vi "Main.vi"() -> ()   [LabVIEW 2018]
doc: "Use this template to build a simple state machine design pattern. Each state executes code and determines which state to transition to."
uses:
  controls/State.ctl
  controls/Data.ctl
  <vilib>/Analysis/NI_AALPro.lvlib
panel:
  in  "mA":dbl=4.0 format="%.3f"
  out "Physical Value":dbl
  in  "Compute Physical Value":bool
  out "Slope":dbl
  out "Offset":dbl
  out "XY Graph":cluster{dbl[], dbl[]}(graph)
  in  "Max mA Output":dbl
  in  "Min mA Output":dbl
  in  "Max Physical Value":dbl
  in  "Min Physical Value":dbl
  in  "Completion Resistor(Ohms)":u16
  in  "Compute Coefficients":bool
  in  "Exit":bool
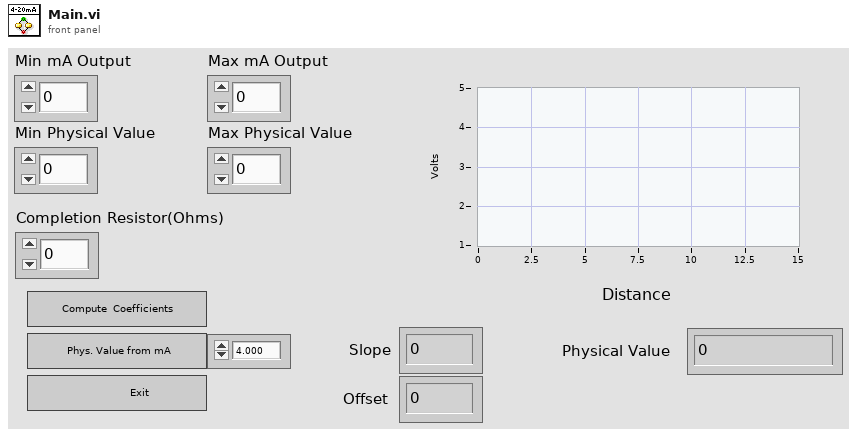
[diagram p1: front panel]
types:
  T1 = typedef "Data.ctl" = cluster{"Completion Resistor(Ohms)":dbl, "Min Physical Value":dbl, "Max Physical Value":dbl, "Min mA Output":dbl, "Max mA Output":dbl, "Measured mA Output":dbl, "Min Voltage":dbl, "Max Voltage":dbl, "m [f(x)]":dbl, "b [f(x)]":dbl, "m [f(y)]":dbl, "b [f(y)]":dbl}
  T2 = typedef "State.ctl" = enum16{"Initialize", "Wait for Event", "Compute Coefficients", "Compute MinMax Volts", "Compute f(x) Slope & Offset", "Compute f(y) Slope & Offset", "Compute Physical Value from mA", "Display Physical Value", "Exit"}
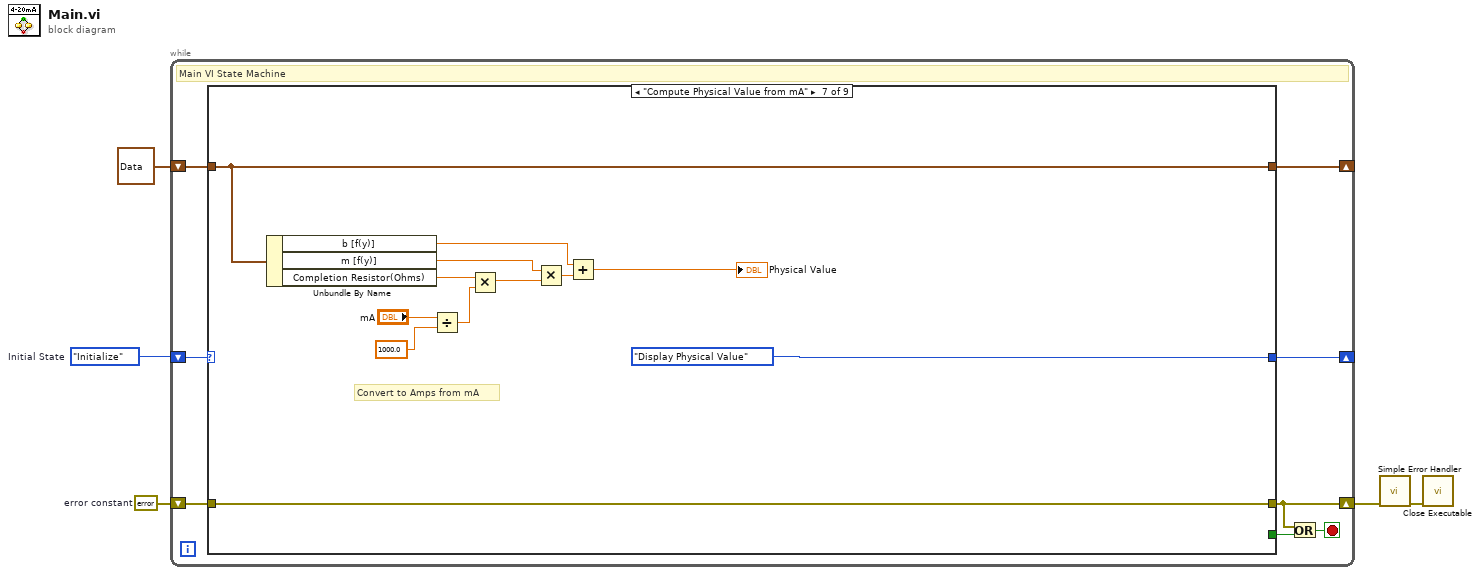
[diagram p0: block diagram]
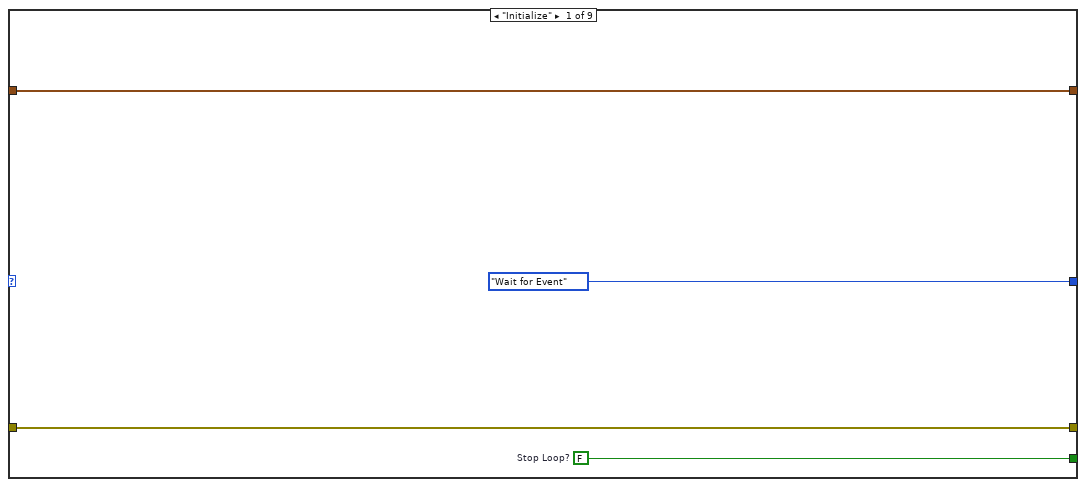
[diagram p2: hidden frame]
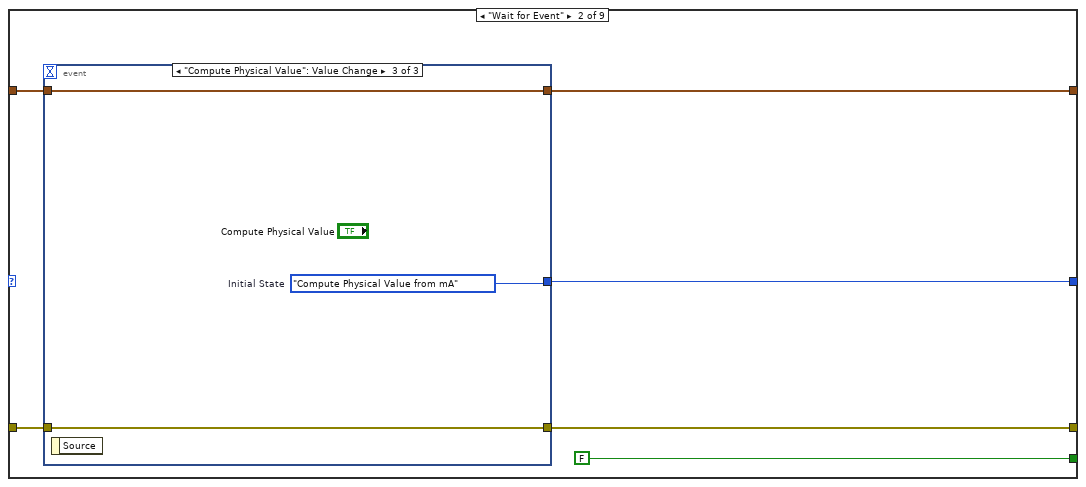
[diagram p3: hidden frame]
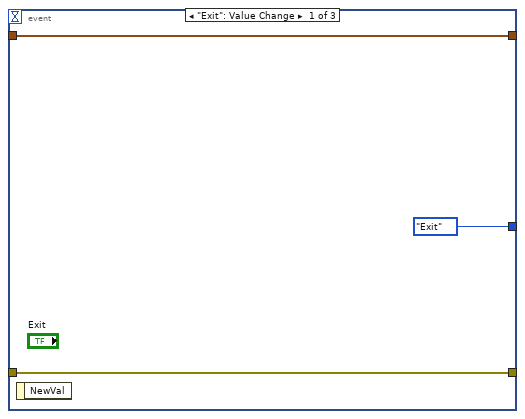
[diagram p4: hidden frame]
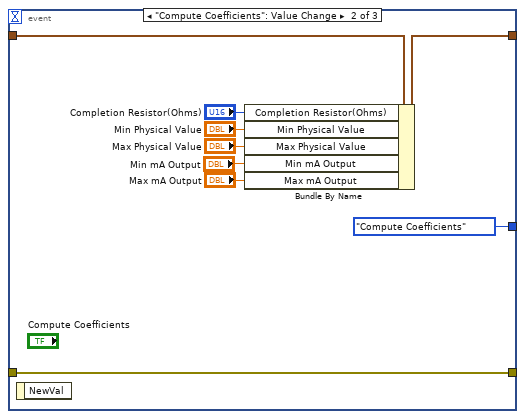
[diagram p5: hidden frame]
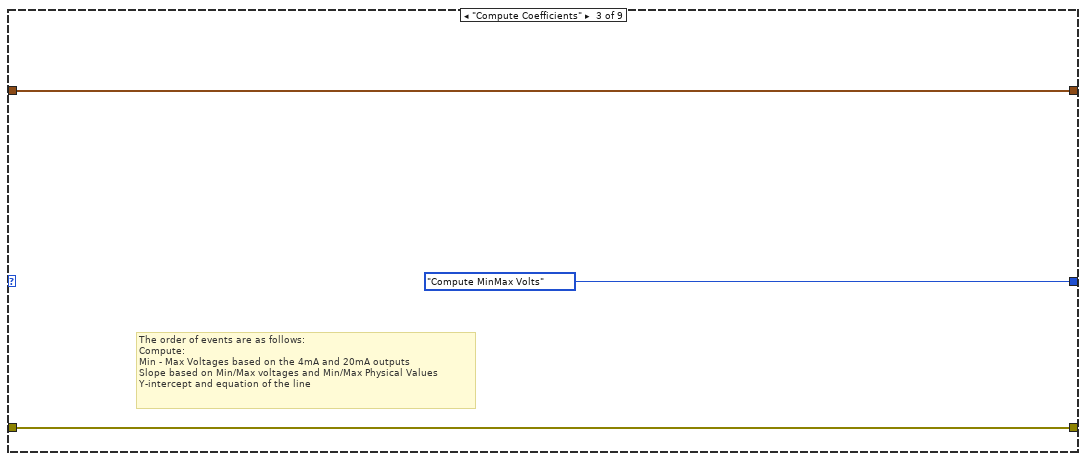
[diagram p6: hidden frame]
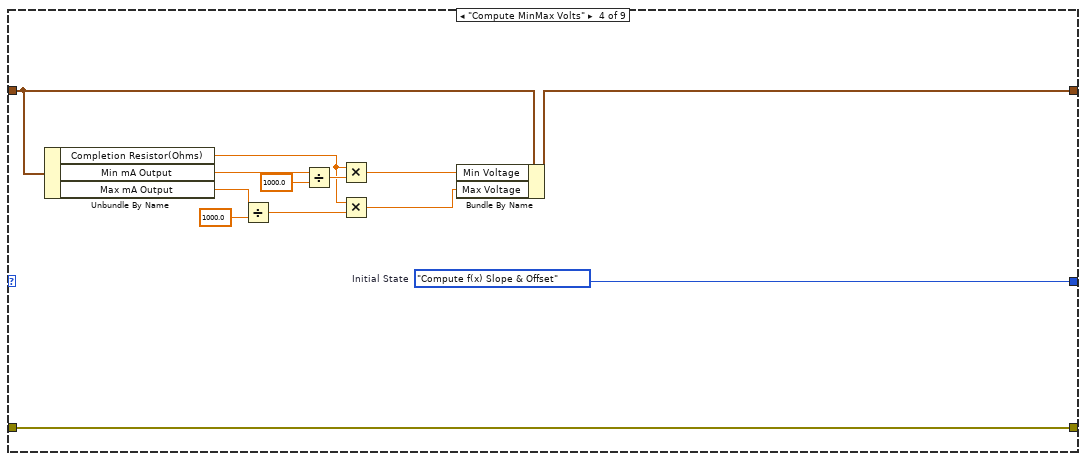
[diagram p7: hidden frame]
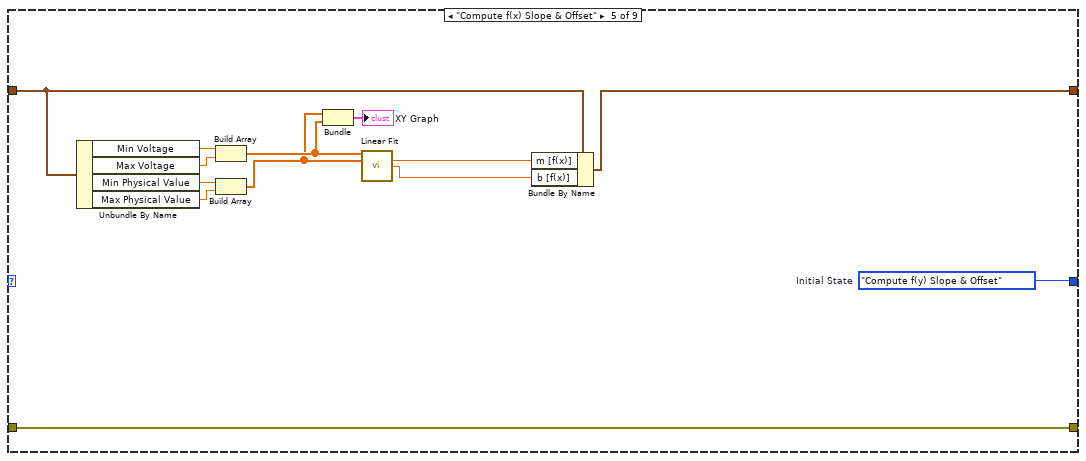
[diagram p8: hidden frame]
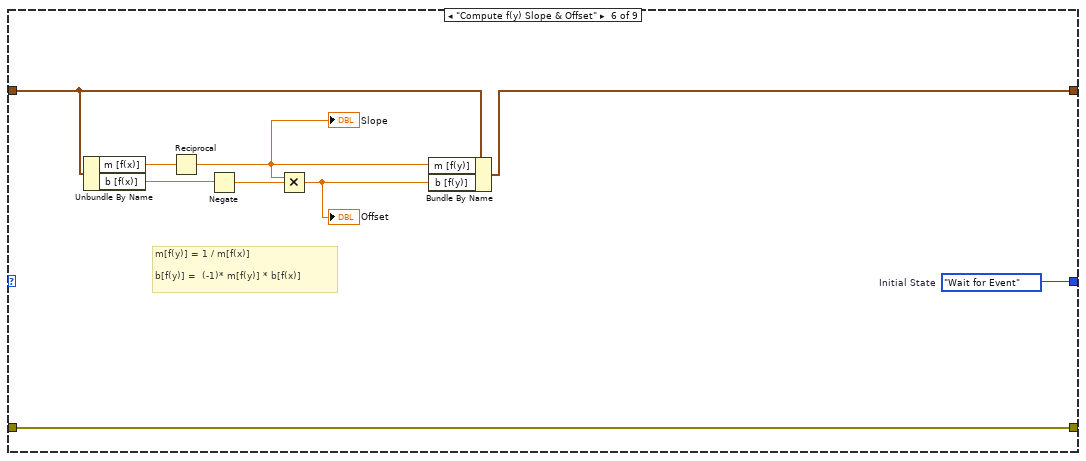
[diagram p9: hidden frame]
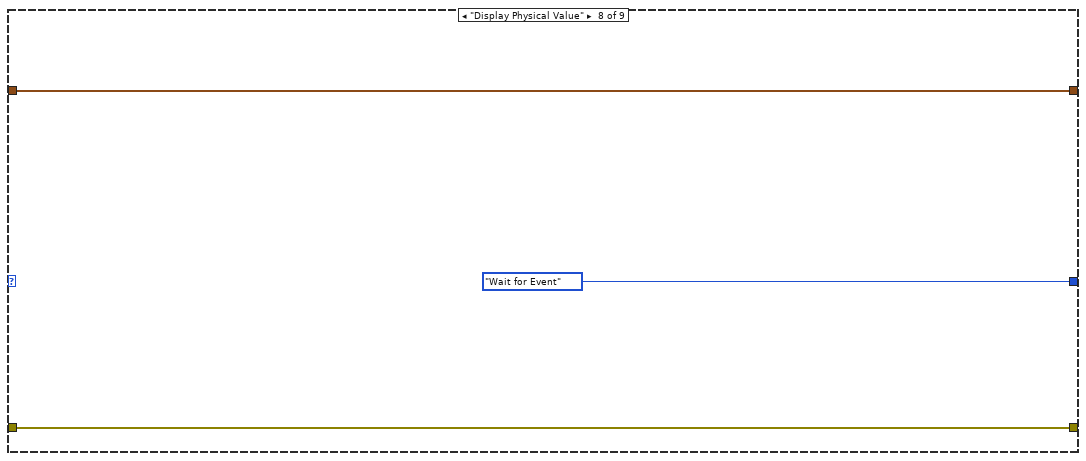
[diagram p10: hidden frame]
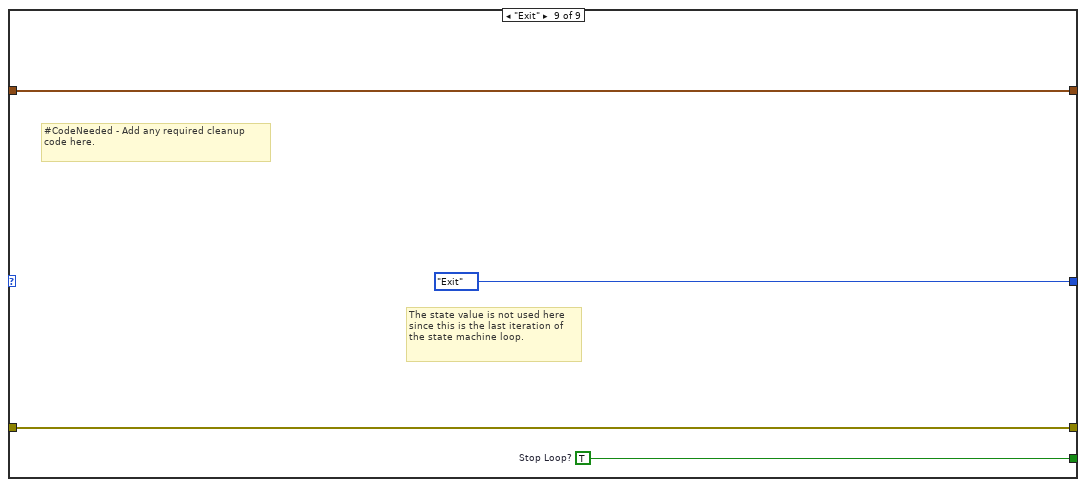
[diagram p11: hidden frame]
diagram:
  w4 = errorcluster {"status"=FALSE, "code"=0, "source"=""}  # error constant
  w1 = State."Initialize"  # Initial State
  n1 = while {
    shift-right: [w6] -> _
    shift-left: w1 -> [w7]
    shift-right: [w12] -> _
    shift-left: T1 {"Completion Resistor(Ohms)"=0.0, "Min Physical Value"=0.0, "Max Physical Value"=0.0, "Min mA Output"=0.0, "Max mA Output"=0.0, "Measured mA Output"=0.0, "Min Voltage"=0.0, "Max Voltage"=0.0, "m [f(x)]"=0.0, "b [f(x)]"=0.0, "m [f(y)]"=0.0, "b [f(y)]"=0.0} ("Data") -> [w13]
    shift-right: [w8] -> w3
    shift-left: w4 -> [w11]
    stop <- w9 stop-if-true
    # "Main VI State Machine"
    n2 = case shown="\"Compute Physical Value from mA\"" w7 {
      tunnel: [State."Wait for Event" ("Next State") w23 State."Compute MinMax Volts" ("Next State") w42 w62 w68 State."Display Physical Value" ("Next State") State."Wait for Event" ("Next State") State."Exit" ("(Value Not Used)")] -> w6
      tunnel: [w16 FALSE ("Stop Loop?") _ _ _ _ _ _ w93] -> w10
      tunnel: w13 -> [w15 w21 w40 w53 w58 w74 w86 w91 w94]
      tunnel: [w15 w20 w40 w52 w55 w73 w86 w91 w94] -> w12
      tunnel: w11 -> [w14 w19 w39 w54 w67 w76 w88 w90 w92]
      tunnel: [w14 w18 w39 w54 w67 w76 w88 w90 w92] -> w8
      frame "Initialize" {
        w16 = FALSE  # Stop Loop?
        # "Initialize - Initialize the application."
      }
      frame "Wait for Event" {
        # "Wait for Event - Use an Event Structure to monitor the user interface for events that run different states of the state machine."
        n3 = event shown="[2] \"Compute Physical Value\": Value Change" {
          selector: _ -> [_ _ _]
          dyn-events: _ -> [_ _ _]
          timeout: _ -> [_ _ _]
          tunnel: [State."Exit" ("Next State") State."Compute Coefficients" ("Next State") w36] -> w23
          tunnel: w21 -> [w25 w35 w38]
          tunnel: [w25 w34 w38] -> w20
          tunnel: w19 -> [w24 w33 w37]
          tunnel: [w24 w33 w37] -> w18
          event "Exit": Value Change {
            n4 = event-data() -> ()  [unwired: 1 in, 1 out]
          }
          event "Compute Coefficients": Value Change {
            n5 = event-data() -> ()  [unwired: 1 in, 1 out]
            n6 = Bundle By Name(cluster=w35, "Completion Resistor(Ohms)"="Completion Resistor(Ohms)", "Min Physical Value"="Min Physical Value", "Max Physical Value"="Max Physical Value", "Min mA Output"="Min mA Output", "Max mA Output"="Max mA Output") -> (w34:T1)
          }
          event "Compute Physical Value": Value Change {
            w36 = State."Compute Physical Value from mA"  # Initial State
            n7 = event-data() -> ()  [unwired: 1 in, 1 out]
          }
        }
      }
      frame "Compute Coefficients" {
        # "The order of events are as follows:\nCompute:\nMin - Max Voltages based on the 4mA and 20mA outputs\nSlope based on Min/Max voltages and Min/Max Physical Values\nY-intercept and equation of the line"
      }
      frame "Compute MinMax Volts" {
        w42 = State."Compute f(x) Slope & Offset"  # Initial State
        n8 = Unbundle By Name(w53) -> ("Completion Resistor(Ohms)"=w43:dbl, "Min mA Output"=w48:dbl, "Max mA Output"=w50:dbl)
        n9 = Divide(x=w50, y=1000.0) -> (x/y=w45:dbl)
        n10 = Divide(x=w48, y=1000.0) -> (x/y=w47:dbl)
        n11 = Multiply(x=w43, y=w47) -> (x*y=w46:dbl)
        n12 = Multiply(x=w43, y=w45) -> (x*y=w44:dbl)
        n13 = Bundle By Name(cluster=w53, "Min Voltage"=w46, "Max Voltage"=w44) -> (w52:T1)
      }
      frame "Compute f(x) Slope & Offset" {
        w62 = State."Compute f(y) Slope & Offset"  # Initial State
        n14 = Unbundle By Name(w58) -> ("Min Voltage"=w66:dbl, "Max Voltage"=w65:dbl, "Min Physical Value"=w64:dbl, "Max Physical Value"=w63:dbl)
        n15 = Build Array(w66, w65) -> (w61:dbl[])
        n16 = Build Array(w64, w63) -> (w60:dbl[])
        n17 = Bundle(w60, w61) -> (→"XY Graph":cluster{dbl[], dbl[]})  [unwired: 1 in]
        n18 = call <vilib>:"Linear Fit.vi"("Y"=w61, "X"=w60) -> ("slope"=w57:dbl, "intercept"=w56:dbl)  [unwired: 9 in, 3 out]
        n19 = Bundle By Name(cluster=w58, "m [f(x)]"=w57, "b [f(x)]"=w56) -> (w55:T1)
      }
      frame "Compute f(y) Slope & Offset" {
        w68 = State."Wait for Event"  # Initial State
        # "m[f(y)] = 1 / m[f(x)]\n\nb[f(y)] =  (-1)* m[f(y)] * b[f(x)]"
        n20 = Unbundle By Name(w74) -> ("m [f(x)]"=w75:dbl, "b [f(x)]"=w72:dbl)
        n21 = Reciprocal(x=w75) -> (1/x=w70:dbl)
        "Slope" <- w70
        n22 = Negate(x=w72) -> (-x=w71:dbl)
        n23 = Multiply(x=w70, y=w71) -> (x*y=w69:dbl)
        "Offset" <- w69
        n24 = Bundle By Name(cluster=w74, "m [f(y)]"=w70, "b [f(y)]"=w69) -> (w73:T1)
      }
      frame "Compute Physical Value from mA" {
        # "Convert to Amps from mA"
        n25 = Unbundle By Name(w86) -> ("b [f(y)]"=w81:dbl, "m [f(y)]"=w84:dbl, "Completion Resistor(Ohms)"=w85:dbl)
        n26 = Divide(x="mA", y=1000.0) -> (x/y=w77:dbl)
        n27 = Multiply(x=w85, y=w77) -> (x*y=w83:dbl)
        n28 = Multiply(x=w84, y=w83) -> (x*y=w82:dbl)
        n29 = Add(x=w81, y=w82) -> (x+y=→"Physical Value":dbl)
      }
      frame "Display Physical Value" {
      }
      frame "Exit" {
        w93 = TRUE  # Stop Loop?
        # "#CodeNeeded - Add any required cleanup code here."
        # "The state value is not used here since this is the last iteration of the state machine loop."
        # "Exit - Exit the application."
      }
    }
    n30 = Or(x=w8, y=w10) -> (x .or. y?=w9:bool)
  }
  n31 = call <vilib>:"Simple Error Handler.vi"("error in (no error)"=w3) -> ("error out"=w2:errorcluster)  [unwired: 4 in, 4 out]
  n32 = call "Close Executable.vi"("error in (no error)"=w2) -> ()  [unwired: 11 in]
